vi "AdderMultiplier.vi"(10 "N2":i64, 11 "N1":i64) -> (2 "Numeric":i64, 3 "Numeric 2":i64)   [LabVIEW 2020]
doc: "This subVI gets two numbers and performs addition and multiplication and gives its output"
panel:
  # "Gets two inputs adds and multiplies it"
  # "INPUT"
  # "OUTPUT"
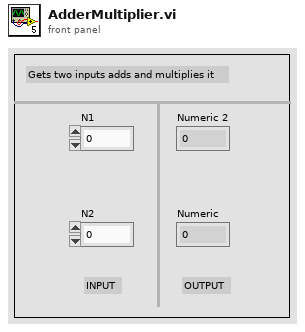
[diagram p1: front panel]
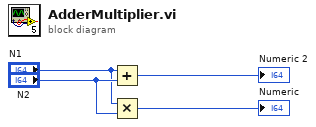
[diagram p0: block diagram]
diagram:
  n1 = Add(x="N1", y="N2") -> (x+y=→"Numeric 2":i64)
  n2 = Multiply(x="N1", y="N2") -> (x*y=→"Numeric":i64)
